vi "Create Progress Bar Events.vi"(8 "error in (no error)":errorcluster, 11 "NI_AB_API_DPPL in":refnum<class "NI_AB_API_DPPL.lvclass">) -> (0 "error out":errorcluster, 2 "progressBarEvents":T1, 3 "NI_AB_API_DPPL out":refnum<class "NI_AB_API_DPPL.lvclass">)   [LabVIEW 2020, in "NI_AB_API_DPPL.lvclass"]
uses:
  <vilib>/AppBuilder/AB_API/DPPL/NI_AB_API_DPPL.lvclass
  <vilib>/AppBuilder/AB_API/DPPL/NI_AB_API_DPPL.lvclass/NI_AB_API_DPPL.ctl
  <vilib>/AppBuilder/AB_API/PPL/NI_AB_API_PPL.lvclass
  <vilib>/AppBuilder/AB_API/common/AB_API ProgressBar_BuildError.ctl
  <vilib>/AppBuilder/AB_API/common/AB_API ProgressBar_Events.ctl
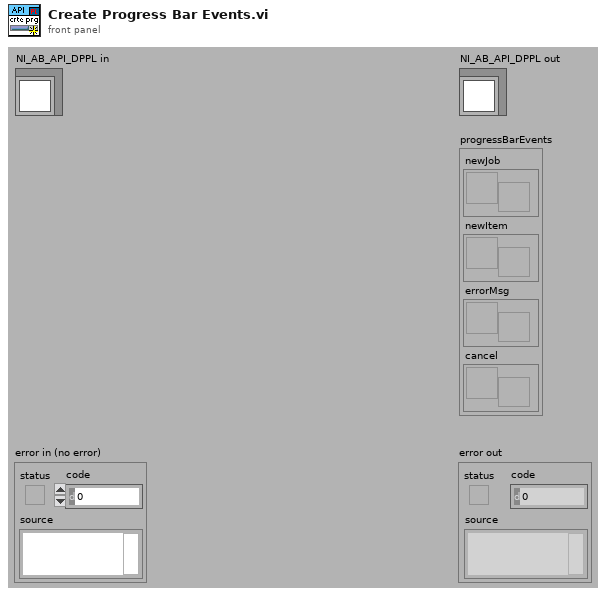
[diagram p1: front panel]
types:
  T1 = typedef "AB_API ProgressBar_Events.ctl" = cluster{"newJob":refnum<user-event>, "newItem":refnum<user-event>, "errorMsg":T2, "cancel":refnum<user-event>}
  T2 = typedef "AB_API ProgressBar_BuildError.ctl" = refnum<user-event>
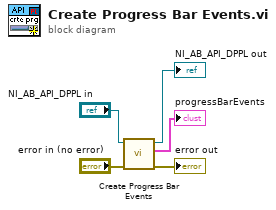
[diagram p0: block diagram]
diagram:
  n1 = call-parent "Create Progress Bar Events.vi"("error in (no error)"="error in (no error)", "NI_AB_API_PPL in"="NI_AB_API_DPPL in") -> ("error out"=→"error out":errorcluster, "progressBarEvents"=→"progressBarEvents":T1, "NI_AB_API_PPL out"=→"NI_AB_API_DPPL out":refnum<class "NI_AB_API_DPPL.lvclass">)  [unwired: 7 in]
